vi "Status String Update.vi"(6 "error in (no error)":errorcluster, 10 "Value":string, 11 "String reference in":refnum<vi>) -> (3 "STring reference out":refnum<vi>)   [LabVIEW 2019]
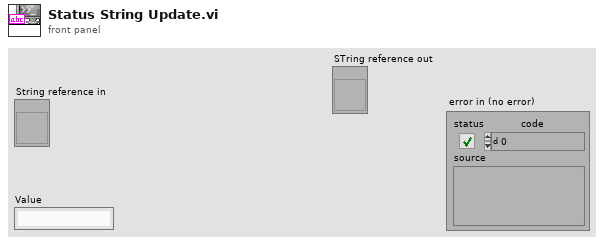
[diagram p1: front panel]
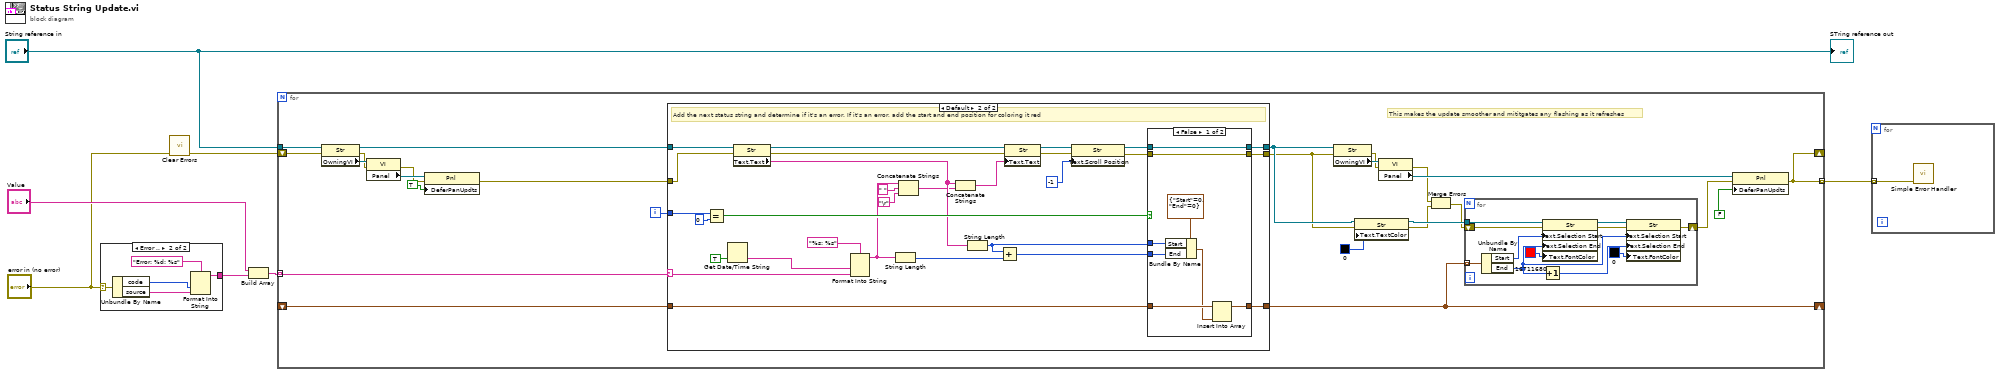
[diagram p0: block diagram]
diagram:
  n1 = case shown="Error .." "error in (no error)" {
    selector: "error in (no error)" -> [_ w12]
    tunnel: [_ w9] -> w5
    frame No Error {
    }
    frame Error {
      n2 = Unbundle By Name(w12) -> ("code"=w10:i32, "source"=w11:string)
      n3 = Format Into String(format string="Error: %d: %s", w10, w11) -> (resulting string=w9:string)  [unwired: 2 in, 1 out]
    }
  }
  n4 = call <vilib>:"Clear Errors.vi"("error in (no error)"="error in (no error)") -> ("error out"=w2:errorcluster)  [unwired: 5 in, 1 out]
  n5 = Build Array("Value", w5) -> (w4:string[])
  n6 = for {
    tunnel: "String reference in" -> [w28]
    tunnel: w4 -> [w38] mode=indexing
    shift-right: [w35] -> _
    shift-left: _ -> [w36]
    shift-right: [w20] -> _
    shift-left: w2 -> [w24]
    tunnel: [w20] -> w1 mode=indexing
    i -> [w37]
    # "This makes the update smoother and mititgates any flashing as it refreshes"
    n7 = property class="Str"(reference=w28, error in=w24) -> (reference out=w27:refnum<vi>, error out=w23:errorcluster, "OwningVI"=w31:refnum<vi>)
    n8 = property class="VI"(reference=w31, error in=w23) -> (error out=w22:errorcluster, "Panel"=w30:refnum<vi>)  [unwired: 1 out]
    n9 = property class="Pnl"(reference=w30, error in=w22, "DeferPanUpdts"=TRUE ("Defer Panel Updates")) -> (error out=w26:errorcluster)  [unwired: 1 out]
    n10 = case shown="Default" w38 {
      selector: w38 -> [_ w70]
      tunnel: w27 -> [w51 w76]
      tunnel: w37 -> [_ w75]
      tunnel: w36 -> [w52 w60]
      tunnel: [w52 w59] -> w35
      tunnel: [w51 w58] -> w18
      tunnel: w26 -> [w50 w57]
      tunnel: [w50 w53] -> w13
      frame "" {
      }
      frame Default {
        # "Add the next status string and determine if it's an error. If it's an error, add the start and end position for coloring it red"
        n11 = Equal?(x=w75, y=0) -> (x = y?=w69:bool)
        n12 = Get Date/Time String(want seconds? (F)=TRUE) -> (time string=w79:string)  [unwired: 2 in, 1 out]
        n13 = property class="Str"(reference=w76, error in=w57) -> (reference out=w62:refnum<vi>, error out=w56:errorcluster, "Text.Text"=w65:string)
        n14 = Format Into String(format string="%s: %s", w79, w70) -> (resulting string=w68:string)  [unwired: 2 in, 1 out]
        n15 = String Length(string=w68) -> (length=w72:i32)
        n16 = Concatenate Strings(w68, " " ("string"), "\r") -> (w64:string)
        n17 = Concatenate Strings(w65, w64) -> (w63:string)
        n18 = String Length(string=w65) -> (length=w73:i32)
        n19 = Add(x=w73, y=w72) -> (x+y=w71:i32)
        n20 = property class="Str"(reference=w62, error in=w56, "Text.Text"=w63) -> (reference out=w61:refnum<vi>, error out=w55:errorcluster)
        n21 = property class="Str"(reference=w61, error in=w55, "Text.Scroll Position"=-1) -> (reference out=w77:refnum<vi>, error out=w54:errorcluster)
        n22 = case shown="False" w69 {
          tunnel: w77 -> [w84 w91]
          tunnel: w73 -> [w89 _]
          tunnel: w71 -> [w88 _]
          tunnel: w60 -> [w87 w92]
          tunnel: [w86 w92] -> w59
          tunnel: [w84 w91] -> w58
          tunnel: w54 -> [w82 w90]
          tunnel: [w82 w90] -> w53
          frame False {
            n23 = Bundle By Name(cluster=cluster{"Start":i32, "End":i32} {"Start"=0, "End"=0}, "Start"=w89, "End"=w88) -> (w85:cluster{"Start":i32, "End":i32})
            n24 = Insert Into Array(array=w87, new element=w85) -> (w86:cluster{"Start":i32, "End":i32}[])  [unwired: 1 in]
          }
          frame True {
          }
        }
      }
    }
    n25 = property class="Str"(reference=w18, error in=w13) -> (error out=w21:errorcluster, "OwningVI"=w34:refnum<vi>)  [unwired: 1 out]
    n26 = property class="Str"(reference=w18, error in=w13, "Text.TextColor"=u32 0 ("Text.Text Colors:Text Color")) -> (reference out=w17:refnum<vi>, error out=w14:errorcluster)
    n27 = property class="VI"(reference=w34, error in=w21) -> (error out=w15:errorcluster, "Panel"=w25:refnum<vi>)  [unwired: 1 out]
    n28 = Merge Errors(w15, w14) -> (w16:errorcluster)
    n29 = for {
      tunnel: w17 -> [w49]
      tunnel: w35 -> [w48] mode=indexing
      shift-right: [w39] -> w32
      shift-left: w16 -> [w41]
      n30 = Unbundle By Name(w48) -> ("Start"=w47:i32, "End"=w42:i32)
      n31 = property class="Str"(reference=w49, error in=w41, "Text.Selection Start"=w47, "Text.Selection End"=w42, "Text.FontColor"=u32 16711680 ("Text.Font:Color")) -> (reference out=w43:refnum<vi>, error out=w40:errorcluster)
      n32 = Increment(x=w42) -> (x+1=w45:i32)
      n33 = property class="Str"(reference=w43, error in=w40, "Text.Selection Start"=w42, "Text.Selection End"=w45, "Text.FontColor"=u32 0 ("Text.Font:Color")) -> (error out=w39:errorcluster)  [unwired: 1 out]
    }
    n34 = property class="Pnl"(reference=w25, error in=w32, "DeferPanUpdts"=FALSE ("Defer Panel Updates")) -> (error out=w20:errorcluster)  [unwired: 1 out]
  }
  n35 = for {
    tunnel: w1 -> [w93] mode=indexing
    n36 = call <vilib>:"Simple Error Handler.vi"("error in (no error)"=w93) -> ()  [unwired: 4 in, 5 out]
  }
  "STring reference out" <- "String reference in"
